vi "DateTimeUTC to TimeDateStamp.vi"(11 "Time String":string="2013-11-25 04:54:00") -> (3 "time stamp":timestamp=timestamp(3468200040 s since 1904-01-01))   [LabVIEW 2012]
uses:
  <vilib>/Utility/miscctls.llb/LVDateTimeRec.ctl
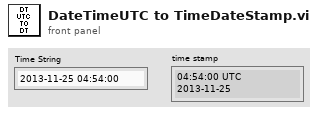
[diagram p1: front panel]
types:
  T1 = typedef "LVDateTimeRec.ctl" = cluster{"fractional second":dbl, "second":i32, "minute":i32, "hour":i32, "day of month":i32, "month":i32, "year":i32, "day of week":i32, "day of year":i32, "DST":i32}
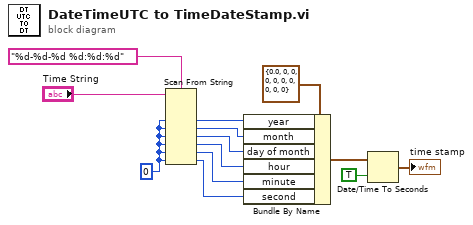
[diagram p0: block diagram]
diagram:
  w7 = 0 ("default value 1")
  n1 = Scan From String(format string="%d-%d-%d %d:%d:%d", input string="Time String", default 1=w7, default 2=w7, default 3=w7, default 4=w7, default 5=w7, default 6=w7) -> (output 1=w6:i32, output 2=w5:i32, output 3=w4:i32, output 4=w3:i32, output 5=w2:i32, output 6=w1:i32)  [unwired: 2 in, 3 out]
  n2 = Bundle By Name(cluster=T1 {"fractional second"=0.0, "second"=0, "minute"=0, "hour"=0, "day of month"=0, "month"=0, "year"=0, "day of week"=0, "day of year"=0, "DST"=0} ("date time rec"), "year"=w6, "month"=w5, "day of month"=w4, "hour"=w3, "minute"=w2, "second"=w1) -> (w10:T1)
  n3 = Date/Time To Seconds(1:TRUE ("is UTC (F)"), 2:w10) -> (0:→"time stamp":timestamp)
